vi "Teleop.vi"(10 "Match Info":T1={"Autonomous Elapsed Seconds"=0.0, "TeleOp Elapsed Seconds"=0.0, "Disabled Elapsed Seconds"=0.0, "Visited Autonomous"=FALSE, "Visited TeleOp"=FALSE, "Visited Disabled"=FALSE, "Autonomous Settings"={"Autonomous Style"=enum."Independent", "VI Refnum"=refnum}}, 11 "Call Context":T2) -> ()   [LabVIEW 2014]
doc: "This VI is called for each TeleOp packet received from the DS where the robot is not disabled. It is often used to read from the joysticks and update I/O or to update setpoints for timed control loops. It should complete and return within 20 milliseconds or it may miss DS packets."
uses:
  <vilib>/Rock Robotics/WPI/DriverStation/WPI_DriverStationDerivedRobotMode.ctl
  <vilib>/Rock Robotics/WPI/DriverStation/WPI_DriverStationMatch Info.ctl
  TypeDefs/Axis Actions.ctl
  TypeDefs/Button Actions.ctl
  TypeDefs/SRE Enum.ctl
  Get Ctrl/Get ctrl Primary Axis.vi
  Get Ctrl/Get ctrl Primary Button.vi
  Robot Global Data.vi
  Get Ctrl/Get ctrl Secondary Button.vi
  Get Ctrl/Get ctrl Secondary axis.vi
panel:
  in  "Open/Close":bool=TRUE
  in  "Robot Arm Location":enum16{"High", "Middle", "Low"}(ring)
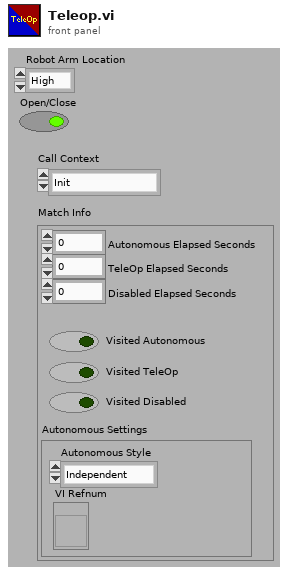
[diagram p1: front panel]
types:
  T1 = typedef "WPI_DriverStationMatch Info.ctl" = cluster{"Autonomous Elapsed Seconds":dbl, "TeleOp Elapsed Seconds":dbl, "Disabled Elapsed Seconds":dbl, "Visited Autonomous":bool, "Visited TeleOp":bool, "Visited Disabled":bool, "Autonomous Settings":cluster{"Autonomous Style":enum16{"Iterative", "Independent"}, "VI Refnum":refnum<vi>}}
  T2 = typedef "WPI_DriverStationDerivedRobotMode.ctl" = enum16{"Init", "Execute", "Stop"}
  T3 = typedef "SRE Enum.ctl" = enum16{"Start", "Run", "End"}
  T4 = enum16{"Auto Stack", "Open/Close claw", "Enable Manuel Elevator", "EM Claw", "Middle Arm", "Middle Lift"}[]
  T5 = typedef "Button Actions.ctl" = enum16{"Toggle Field Centric", "Gyro Reset", "Clear Faults", "Reduce Speed", "Output"}
  T6 = typedef "Axis Actions.ctl" = enum16{"Translate X", "Translate Y", "Rotate"}
  T7 = enum16{"manual Control of arm", "manual Control of Elevator", "Output Control"}[]
  T8 = cluster{"TranslateX":dbl, "TranslateY":dbl, "Rotate":dbl}
  T9 = cluster{"Speed":dbl, "Direction":dbl, "Rotation":dbl}
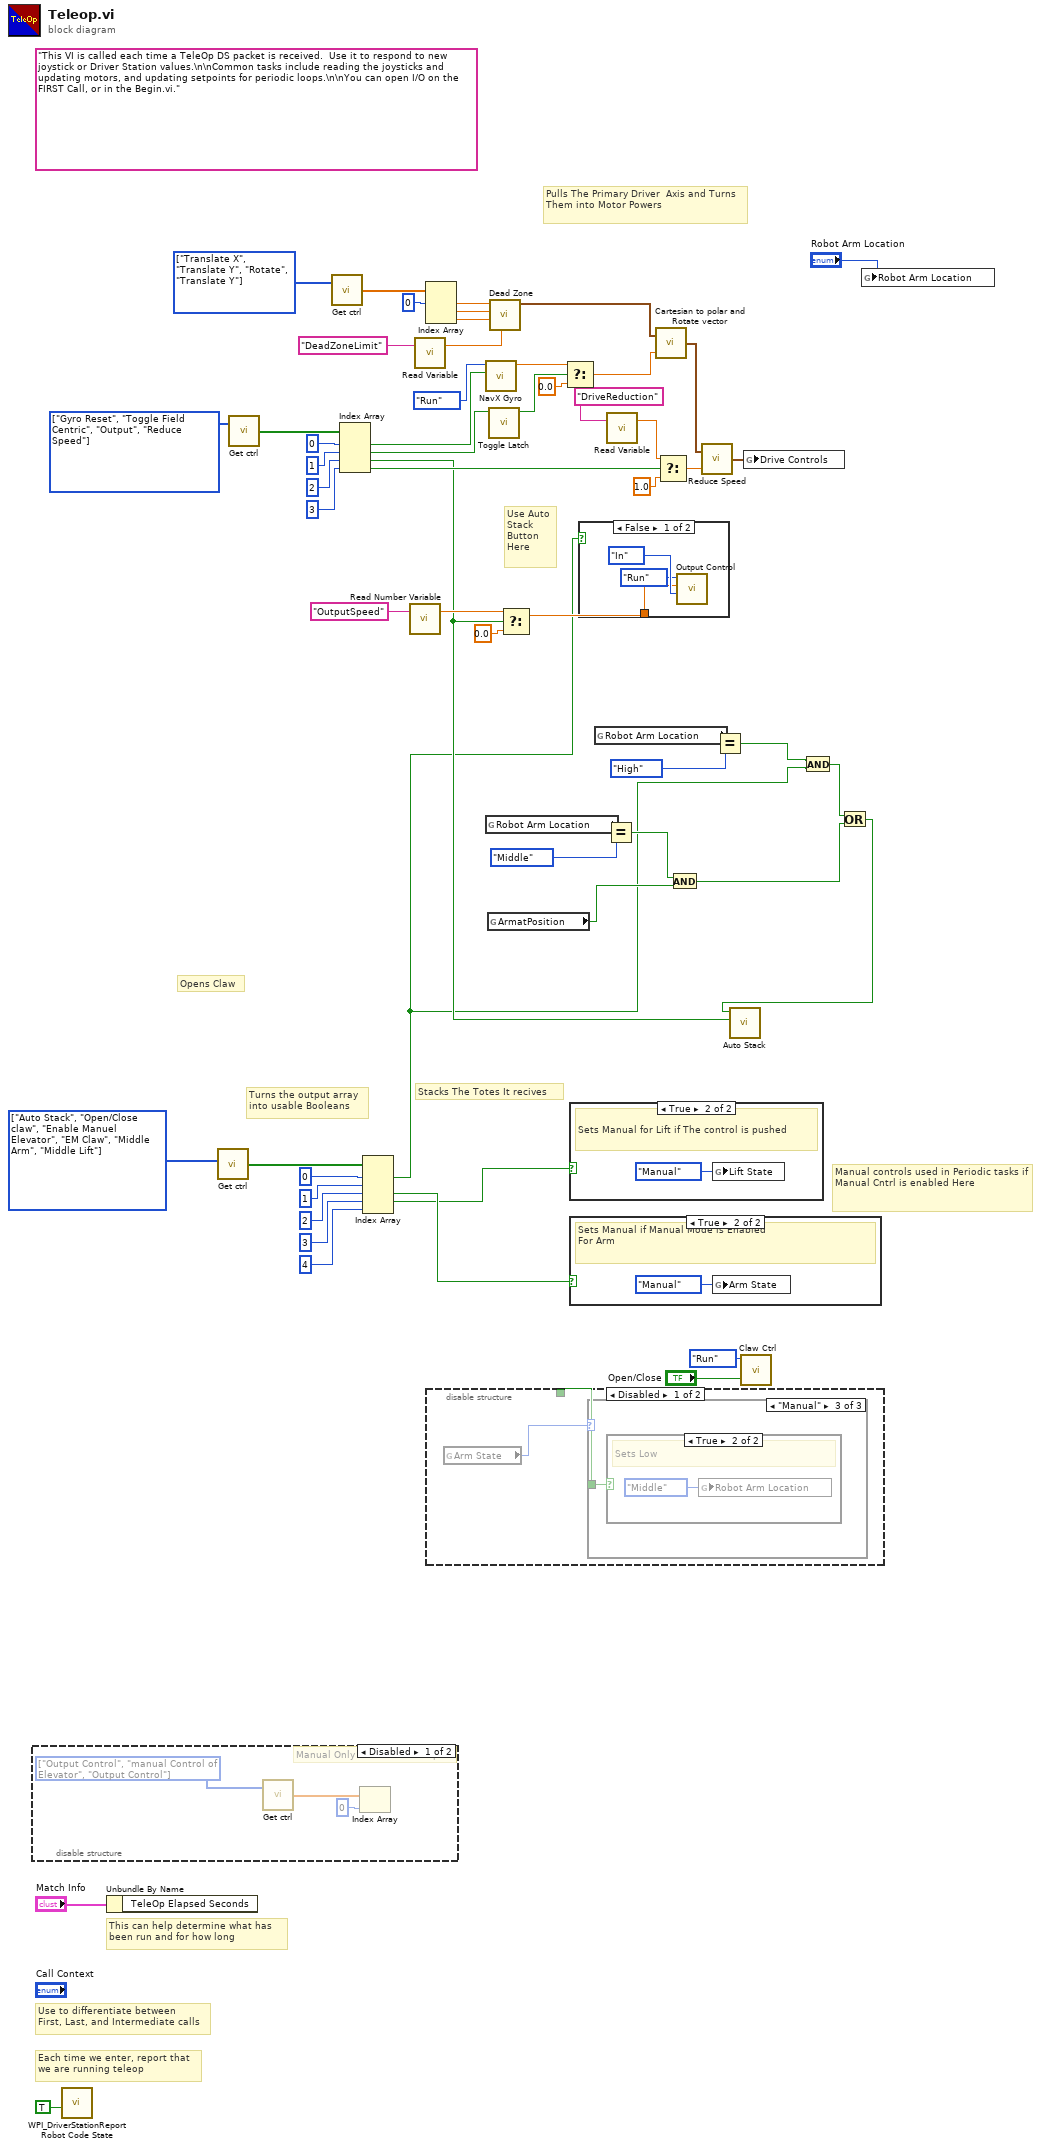
[diagram p0: block diagram]
diagram:
  w18 = T4 [enum."Auto Stack", enum."Open/Close claw", enum."Enable Manuel Elevator", enum."EM Claw", enum."Middle Arm", enum."Middle Lift"] items=["Auto Stack", "Open/Close claw", "Enable Manuel Elevator", "EM Claw", "Middle Arm", "Middle Lift"] ("Controls")
  w26 = T5[] [enum."Gyro Reset", enum."Toggle Field Centric", enum."Output", enum."Reduce Speed"] items=["Toggle Field Centric", "Gyro Reset", "Clear Faults", "Reduce Speed", "Output"] ("Controls")
  w48 = T6[] [enum."Translate X", enum."Translate Y", enum."Rotate", enum."Translate Y"] items=["Translate X", "Translate Y", "Rotate"]
  (unwired) "This VI is called each time a TeleOp DS packet is received.  Use it to respond to new joystick or Driver Station values.\n\nCommon tasks include reading the joysticks and updating motors, and updating setpoints for periodic loops.\n\nYou can open I/O on the FIRST Call, or in the Begin.vi."
  # "Use Auto\nStack\nButton\nHere"
  # "Stacks The Totes It recives"
  # "Opens Claw"
  # "Manual controls used in Periodic tasks if Manual Cntrl is enabled Here"
  # "Turns the output array\ninto usable Booleans"
  # "Pulls The Primary Driver  Axis and Turns Them into Motor Powers"
  # "Each time we enter, report that\nwe are running teleop"
  # "Use to differentiate between\nFirst, Last, and Intermediate calls"
  # "This can help determine what has\nbeen run and for how long"
  n1 = disable-structure shown="Disabled" {
    frame Disabled {
      w62 = T7 [enum."Output Control", enum."manual Control of Elevator", enum."Output Control"] items=["manual Control of arm", "manual Control of Elevator", "Output Control"] ("TypeDef")
      # "Manual Only for use in Teleop"
      n2 = call-poly "Get ctrl.vi"("TypeDef"=w62) -> ("Array"=w61:dbl[])  [unwired: 2 in]
      n3 = Index Array(array=w61, index=0) -> ()  [unwired: 1 out]
    }
    frame Enabled {
    }
  }
  n4 = call <vilib>:"WPI_DriverStationReport Robot Code State.vi"("TeleOp"=TRUE ("Autonomous")) -> ()  [unwired: 10 in, 1 out]
  n5 = Unbundle By Name("Match Info") -> ()  [unwired: 1 out]
  n6 = call-poly "Get ctrl.vi"("Controls"=w18) -> ("Array"=w24:bool[])  [unwired: 2 in]
  n7 = call-poly "Get ctrl.vi"("Controls"=w26) -> ("Output"=w45:bool[])  [unwired: 2 in]
  n8 = call-poly "Get ctrl.vi"("Controls"=w48) -> ("Axes"=w46:dbl[])  [unwired: 2 in]
  n9 = Index Array(array=w45, index #1=0 ("index"), index #2=1 ("index"), index #3=2 ("index"), index #4=3 ("index")) -> (element #1=w41:bool, element #2=w40:bool, element #3=w14:bool, element #4=w25:bool)
  n10 = Index Array(array=w24, index #1=0 ("index"), index #2=1 ("index"), index #3=2 ("index"), index #4=3 ("index"), index #5=4 ("index")) -> (element #1=w4:bool, element #3=w17:bool, element #4=w16:bool)  [unwired: 2 out]
  n11 = call "Read Number Variable.vi"("Name"="OutputSpeed") -> ("number"=w33:dbl)  [unwired: 1 in, 1 out]
  n12 = call-poly "Read Variable.vi"("Name"="DeadZoneLimit") -> ("number"=w35:dbl)  [unwired: 1 in, 1 out]
  n13 = Index Array(array=w46, index #1=0 ("index")) -> (element #1=w39:dbl, element #2=w38:dbl, element #3=w37:dbl)  [unwired: 2 in]
  n14 = disable-structure shown="Disabled" {
    disable-tunnel: _ -> [w63 _]
    frame Disabled {
      n15 = global read "Robot Global Data.vi" "Arm State"() -> (w64:enum16{"Initializing", "Running", "Manual"})
      n16 = case shown="\"Manual\"" w64 {
        tunnel: w63 -> [_ _ w65]
        frame "Initializing", Default {
        }
        frame "Running" {
        }
        frame "Manual" {
          n17 = case shown="True" w65 {
            frame False {
            }
            frame True {
              # "Sets Low"
              n18 = global write "Robot Global Data.vi" "Robot Arm Location"(enum16{"High", "Middle", "Low"}."Middle" ("Robot Arm Location")) -> ()
            }
          }
        }
      }
    }
    frame Enabled {
    }
  }
  n19 = call "NavX Gyro.vi"("Reset"=w41, "Enum"=SRE_Enum."Run") -> ("Angle"=w56:dbl)  [unwired: 8 in, 1 out]
  n20 = global read "Robot Global Data.vi" "Robot Arm Location"() -> (w11:enum16{"High", "Middle", "Low"})
  n21 = global read "Robot Global Data.vi" "ArmatPosition"() -> (w6:bool)
  n22 = call "Toggle Latch.vi"("Clamp Toggled?"=w40) -> ("Clamp Toggled"=w54:bool)  [unwired: 10 in]
  n23 = call "Dead Zone.vi"("Dead Zone limit"=w35, "Rotate"=w37, "TranslateY"=w38, "TranslateX"=w39) -> ("Cluster"=w29:T8)  [unwired: 5 in]
  n24 = Select(t=w33, s=w14, f=0.0) -> (s? t:f=w31:dbl)
  n25 = Select(t=w56, s=w54, f=0.0) -> (s? t:f=w28:dbl)
  n26 = case shown="True" w16 {
    frame False {
    }
    frame True {
      # "Sets Manual for Lift if The control is pushed"
      n27 = global write "Robot Global Data.vi" "Lift State"(enum16{"Initializing", "Running", "Manual"}."Manual" ("Lift State")) -> ()
    }
  }
  n28 = case shown="True" w17 {
    frame False {
    }
    frame True {
      # "Sets Manual if Manual Mode is Enabled\nFor Arm"
      n29 = global write "Robot Global Data.vi" "Arm State"(enum16{"Initializing", "Running", "Manual"}."Manual" ("Lift State")) -> ()
    }
  }
  n30 = case shown="False" w4 {
    tunnel: w31 -> [w69 _]
    frame False {
      n31 = call "Output Control.vi"("Direction"=enum16{"In", "Out", "Done"}."In", "Power"=w69, "Mode"=SRE_Enum."Run") -> ()  [unwired: 9 in]
    }
    frame True {
    }
  }
  n32 = global read "Robot Global Data.vi" "Robot Arm Location"() -> (w8:enum16{"High", "Middle", "Low"})
  n33 = Equal?(x=w11, y=enum16{"High", "Middle", "Low"}."Middle") -> (x = y?=w7:bool)
  n34 = call-poly "Read Variable.vi"("Name"="DriveReduction") -> ("number"=w49:dbl)  [unwired: 1 in, 1 out]
  n35 = call "Cartesian to polar and Rotate vector.vi"("Angle"=w28, "Cluster"=w29) -> ("output cluster"=w27:T9)
  n36 = Select(t=w49, s=w25, f=1.0) -> (s? t:f=w52:dbl)
  n37 = And(x=w7, y=w6) -> (x .and. y?=w2:bool)
  n38 = call "Reduce Speed.vi"("Reduction Factor"=w52, "Drive Controls"=w27) -> ("Drive Controls"=w53:T9)
  n39 = Equal?(x=w8, y=enum16{"High", "Middle", "Low"}."High") -> (x = y?=w5:bool)
  n40 = call "Claw Ctrl.vi"("Open/Close"="Open/Close", "Enum"=SRE_Enum."Run") -> ()  [unwired: 10 in]
  n41 = global write "Robot Global Data.vi" "Drive Controls"(w53) -> ()
  n42 = And(x=w5, y=w4) -> (x .and. y?=w3:bool)
  n43 = Or(x=w3, y=w2) -> (x .or. y?=w1:bool)
  n44 = call "Auto Stack.vi"("Reset Tote Count"=w14, "Use Auto Stack"=w1) -> ()  [unwired: 9 in, 1 out]
  n45 = global write "Robot Global Data.vi" "Robot Arm Location"("Robot Arm Location") -> ()
